vi "Untitled 2.vi"() -> ()   [LabVIEW 2022 SP3]
panel:
  out "x-y*floor(x/y)":i32
  in  "y":i32=100
  in  "x":i32
  out "floor(x/y)":i32
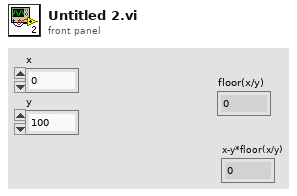
[diagram p1: front panel]
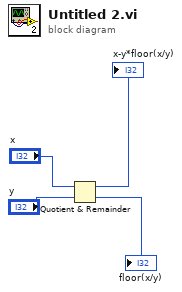
[diagram p0: block diagram]
diagram:
  n1 = Quotient & Remainder(x="x", y="y") -> (x-y*floor(x/y)=→"x-y*floor(x/y)":i32, floor(x/y)=→"floor(x/y)":i32)
